vi "Stop Children.vi"(11 "ActorMeter in":refnum<class "ActorMeter.lvclass">) -> ()   [LabVIEW 2014, in "ActorMeter.lvclass"]
uses:
  ActorMeter.lvclass
  ActorMeter.lvclass/ActorMeter.ctl
  <vilib>/ActorFramework/Stop Msg/Stop Msg.lvclass/Stop Msg.ctl
  <vilib>/ActorFramework/Message Enqueuer/Message Enqueuer.lvclass/Message Enqueuer.ctl
  <vilib>/ActorFramework/Message Enqueuer/Enqueue Critical.vi
  <vilib>/ActorFramework/Message Priority Queue/Priority Enqueue.vi
  <vilib>/ActorFramework/Stop Msg/Stop Msg.lvclass
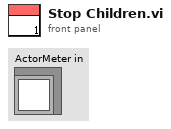
[diagram p1: front panel]
types:
  T1 = cluster{"ReadoutDevice":refnum<class "Message Enqueuer.lvclass">, "ParameterDevice":refnum<class "Message Enqueuer.lvclass">, "Processor":refnum<class "Message Enqueuer.lvclass">, "Collector":refnum<class "Message Enqueuer.lvclass">, "Extractor":refnum<class "Message Enqueuer.lvclass">, "ExperimentService":refnum<class "Message Enqueuer.lvclass">, "StorageService":refnum<class "Message Enqueuer.lvclass">}
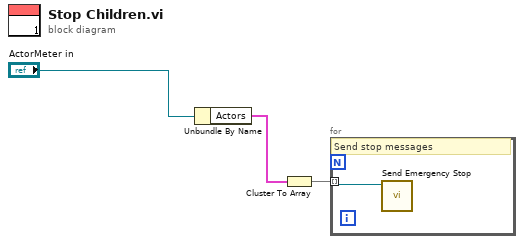
[diagram p0: block diagram]
diagram:
  n1 = Unbundle By Name("ActorMeter in") -> ("Actors"=w2:T1)
  n2 = Cluster To Array(cluster=w2) -> (array=w3:refnum<class "Message Enqueuer.lvclass">[])
  n3 = for {
    tunnel: w3 -> [w4] mode=indexing
    # "Send stop messages"
    n4 = call <vilib>:"Send Emergency Stop.vi"("Message Enqueuer"=w4) -> ()  [unwired: 10 in, 1 out]
  }
